vi "Get Module Block Data Refs.vi"(8 "error in":errorcluster, 9 "Device Ref in":T2 format="%.0x", 11 "Item Ref in":T2 format="%.0x") -> (0 "error out":errorcluster, 1 "Output Data":dbl[](array[numeric]), 2 "Output Block Data Refs":T3[](array[typedef]) {"Data Reference" format="%.0x"}, 3 "Item Ref out":T2=18446744073709551615 format="%.0x", 4 "Input Data":dbl[](array[numeric]), 5 "Mixed IO":T1, 6 "Input Block Data Refs":T3[](array[typedef]) {"Data Reference" format="%.0x"})   [LabVIEW 2019, in "Scan Engine Custom Device.lvlib"]
uses:
  Scan Engine Custom Device.lvlib
  <vilib>/NI VeriStand/Custom Device API/Custom Device Channel Type.ctl
  <vilib>/NI VeriStand/Custom Device API/Custom Device API.lvlib
  <vilib>/NI VeriStand/Custom Device API/Data Access Type.ctl
  Type Defs/Mixed IO.ctl
  <vilib>/NI VeriStand/Custom Device API/Get Item Property (U16).vi
  Modules.lvlibp/RSI Module/Class Property Strings.vi
  <vilib>/NI VeriStand/Custom Device API/Data Reference.ctl
  <vilib>/NI VeriStand/Custom Device API/Block Data Reference.ctl
  <vilib>/NI VeriStand/Custom Device API/Custom Device Item Ref.ctl
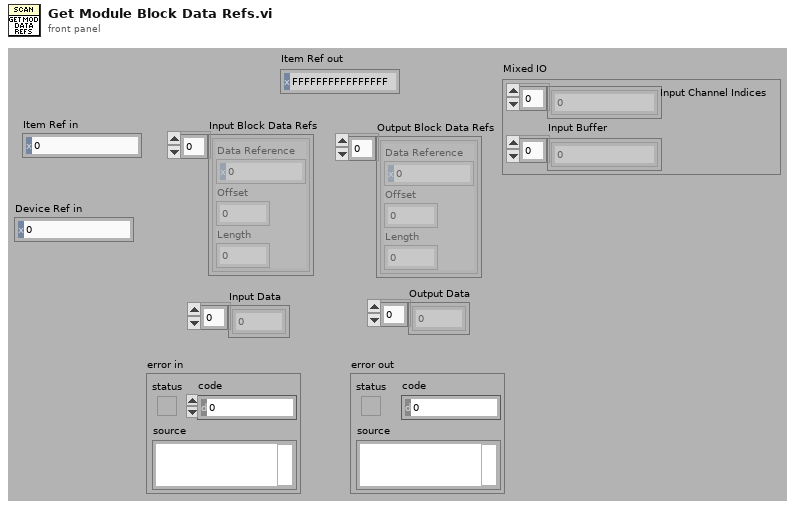
[diagram p1: front panel]
types:
  T1 = typedef "Scan Engine Custom Device.lvlib/Mixed IO.ctl" = cluster{"Input Channel Indices":i32[], "Input Buffer":dbl[]}
  T2 = typedef "Custom Device API.lvlib/Custom Device Item Ref.ctl" = u64
  T3 = typedef "Custom Device API.lvlib/Block Data Reference.ctl" = cluster{"Data Reference":T4, "Offset":u64, "Length":u64}
  T4 = typedef "Custom Device API.lvlib/Data Reference.ctl" = i32
  T5 = typedef "Custom Device API.lvlib/Custom Device Channel Type.ctl" = enum16{"Input", "Output"}
  T6 = typedef "Custom Device API.lvlib/Data Access Type.ctl" = enum16{"Read", "Write"}
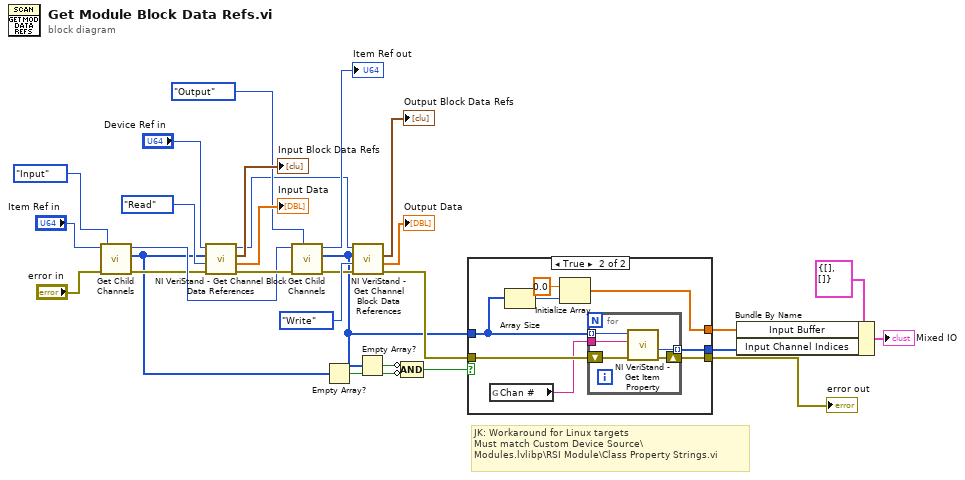
[diagram p0: block diagram]
diagram:
  # "JK: Workaround for Linux targets\nMust match Custom Device Source\\\nModules.lvlibp\\RSI Module\\Class Property Strings.vi"
  n1 = call "Get Child Channels.vi"("Channel Type"=Custom_Device_Channel_Type."Input", "error in"="error in", "Section Ref in"="Item Ref in") -> ("error out"=w13:errorcluster, "Channel Refs"=w11:T2[], "Section Ref out"=w14:T2)  [unwired: 5 in, 1 out]
  n2 = call <vilib>:"NI VeriStand - Get Channel Block Data References.vi"("error in (no error)"=w13, "Access"=Data_Access_Type."Read", "Channel Refs"=w11, "Device Ref in"="Device Ref in") -> ("error out"=w18:errorcluster, "Values Array"=→"Input Data":dbl[], "Block Data Refs"=→"Input Block Data Refs":T3[], "Device Ref out"=w17:T2)  [unwired: 4 in]
  n3 = call "Get Child Channels.vi"("Channel Type"=Custom_Device_Channel_Type."Output", "error in"=w18, "Section Ref in"=w14) -> ("error out"=w19:errorcluster, "Channel Refs"=w7:T2[], "Section Ref out"=→"Item Ref out":T2)  [unwired: 5 in, 1 out]
  n4 = Empty Array?(array=w11) -> (empty?=w10:bool)
  n5 = call <vilib>:"NI VeriStand - Get Channel Block Data References.vi"("error in (no error)"=w19, "Access"=Data_Access_Type."Write", "Channel Refs"=w7, "Device Ref in"=w17) -> ("error out"=w8:errorcluster, "Values Array"=→"Output Data":dbl[], "Block Data Refs"=→"Output Block Data Refs":T3[])  [unwired: 4 in, 1 out]
  n6 = Empty Array?(array=w7) -> (empty?=w9:bool)
  n7 = Compound Arithmetic op=AND(invert w9, invert w10) -> (w2:bool)
  n8 = case shown="True" w2 {
    tunnel: w8 -> [w29 w37]
    tunnel: w7 -> [_ w34]
    tunnel: [_ w36] -> w5
    tunnel: [w29 w35] -> w3
    tunnel: [_ w31] -> w1
    frame False {
    }
    frame True {
      n9 = global read "Class Property Strings.vi" "Chan #"() -> (w30:string)
      n10 = Array Size(array=w34) -> (size(s)=w33:i32)
      n11 = Initialize Array(0.0, w33) -> (w31:dbl[])
      n12 = for {
        tunnel: w34 -> [w41] mode=indexing
        tunnel: [w40] -> w36 mode=indexing
        shift-right: [w39] -> w35
        shift-left: w37 -> [w42]
        tunnel: w30 -> [w38]
        n13 = call-poly <vilib>:"NI VeriStand - Get Item Property.vi"("error in (no error)"=w42, "Property Name"=w38, "Item Ref in"=w41) -> ("error out"=w39:errorcluster, "Value"=w40:u16)  [unwired: 5 in, 2 out]
      }
    }
  }
  "error out" <- w3
  n14 = Bundle By Name(cluster=T1 {"Input Channel Indices"=[], "Input Buffer"=[]} ("Mixed IO"), "Input Buffer"=w1, "Input Channel Indices"=w5) -> (→"Mixed IO":T1)
